vi "FilterMetrics.vi"(11 "supported metrics":string[](array[string])) -> (2 "startup metrics":string[](array[string]), 3 "low-rate supported metrics":string[](array[string]))   [LabVIEW 2017, in "McsaAnalysisLowRate.lvlib"]
uses:
  <vilib>/addons/InsightCM/Devices/Shared/Mcsa/McsaAnalysisLowRate/McsaAnalysisLowRate.lvlib
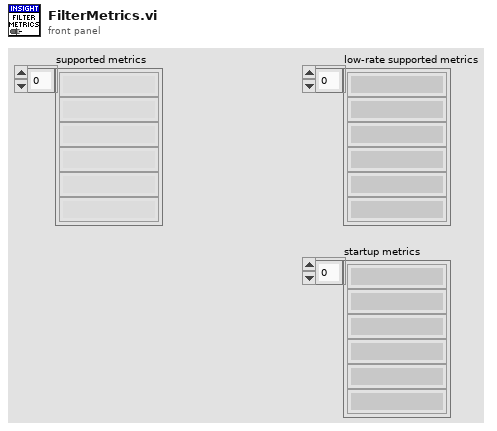
[diagram p1: front panel]
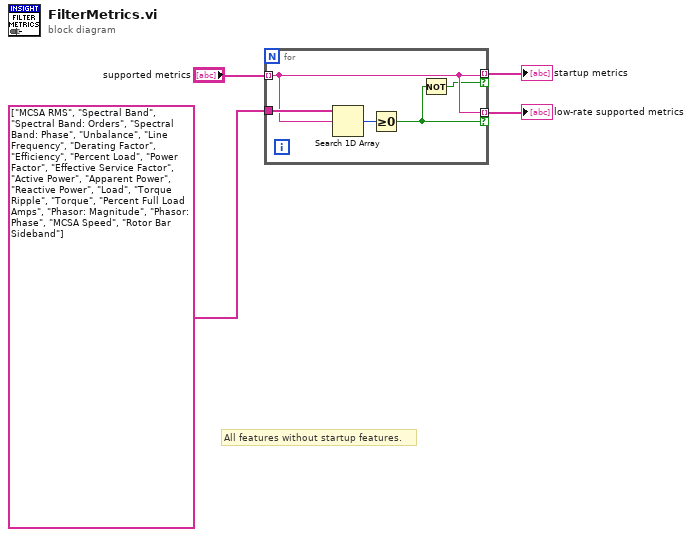
[diagram p0: block diagram]
diagram:
  # "All features without startup features."
  n1 = for {
    tunnel: "supported metrics" -> [w7] mode=indexing
    tunnel: string[] ["MCSA RMS", "Spectral Band", "Spectral Band: Orders", "Spectral Band: Phase", "Unbalance", "Line Frequency", "Derating Factor", "Efficiency", "Percent Load", "Power Factor", "Effective Service Factor", "Active Power", "Apparent Power", "Reactive Power", "Load", "Torque Ripple", "Torque", "Percent Full Load Amps", "Phasor: Magnitude", "Phasor: Phase", "MCSA Speed", "Rotor Bar Sideband"] ("value") -> [w9]
    tunnel: [w7] -> w3 mode=indexing if=w6
    tunnel: [w7] -> w1 mode=indexing if=w5
    n2 = Search 1D Array(1D array=w9, element=w7) -> (index of element=w8:i32)  [unwired: 1 in]
    n3 = Greater Or Equal To 0?(x=w8) -> (x >= 0?=w6:bool)
    n4 = Not(x=w6) -> (.not. x?=w5:bool)
  }
  "low-rate supported metrics" <- w3
  "startup metrics" <- w1
